vi "Error Handler - Event Handling Loop.vi"(8 "error in (no error)":cluster{"状态":bool, "代码":i32, "源":string} caption="错误输入（无错误）", 10 "忽略错误（运行时）":i32[](array[numeric]), 11 "消息队列":refnum<queue>) -> (0 "错误输入副本":cluster{"状态":bool, "代码":i32, "源":string}, 3 "消息队列副本":refnum<queue>)   [LabVIEW 2018]
doc: "对“事件处理循环”中出现的错误进行处理：忽略该错误，或者为该错误生成一个Error消息。"
uses:
  Message Queue/Message Cluster.ctl
  Message Queue/Message Queue.lvlib
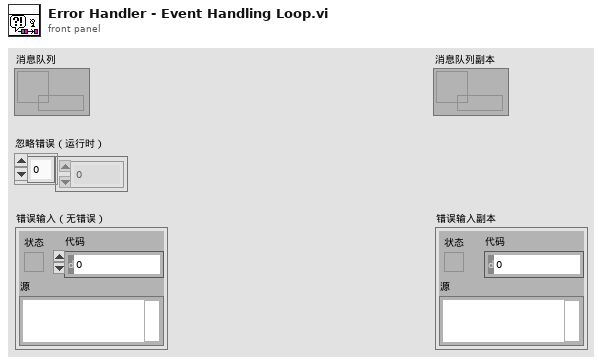
[diagram p1: front panel]
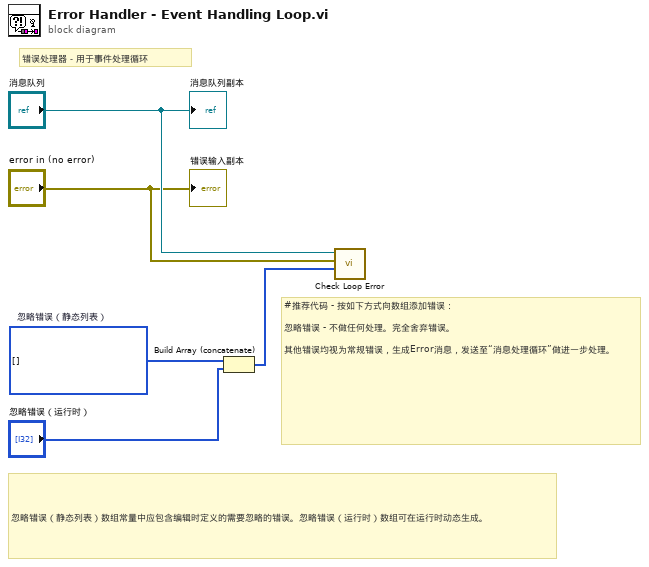
[diagram p0: block diagram]
diagram:
  w4 = i32[] []  # 忽略错误（静态列表）
  # "忽略错误（静态列表）数组常量中应包含编辑时定义的需要忽略的错误。忽略错误（运行时）数组可在运行时动态生成。"
  # "#推荐代码 - 按如下方式向数组添加错误：\n\n忽略错误 - 不做任何处理。完全舍弃错误。\n\n其他错误均视为常规错误，生成Error消息，发送至“消息处理循环”做进一步处理。"
  # "错误处理器－用于事件处理循环"
  n1 = Build Array (concatenate)(w4, "忽略错误（运行时）") -> (w3:i32[])
  n2 = call "Check Loop Error.vi"("忽略错误"=w3, "待处理的错误"="error in (no error)", "消息队列"="消息队列") -> ()  [unwired: 7 in, 2 out]
  "消息队列副本" <- "消息队列"
  "错误输入副本" <- "error in (no error)"
